vi "Note Result.vi"(8 "error in (no error)":errorcluster, 10 "Acquired Result.lvclass":refnum<class "Acquired Result.lvclass">, 11 "Measure Controller in":refnum<class "Measure Controller.lvclass">) -> (0 "error out":errorcluster, 3 "Measure Controller out":refnum<class "Measure Controller.lvclass">)   [LabVIEW 2015, in "Measure Controller.lvclass"]
uses:
  Measure Controller.lvclass
  Results/Acquired Result/Acquired Result.lvclass
  Results/Acquired Result/Acquired Result.lvclass/Acquired Result.ctl
  Measure Controller.lvclass/Measure Controller.ctl
  Results/Acquired Result/Read Sender.vi
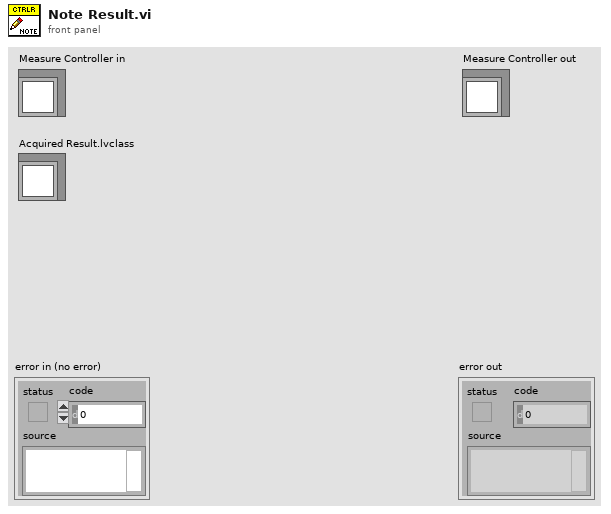
[diagram p1: front panel]
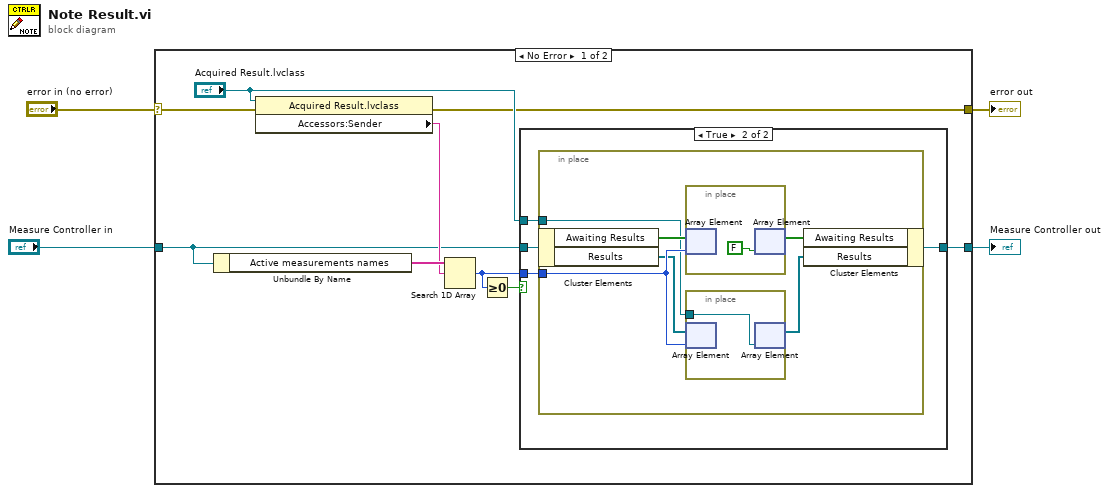
[diagram p0: block diagram]
diagram:
  n1 = case shown="No Error" "error in (no error)" {
    selector: "error in (no error)" -> [w10 w28]
    tunnel: [w9 w28] -> w3
    tunnel: [w7 w27] -> w1
    tunnel: "Measure Controller in" -> [w8 w27]
    frame No Error {
      n2 = Unbundle By Name(w8) -> ("Active measurements names"=w13:string[])
      n3 = property class="Acquired Result.lvclass"(reference="Acquired Result.lvclass", error in=w10) -> (error out=w9:errorcluster, "Accessors:Sender"=w12:string)  [unwired: 1 out]
      n4 = Search 1D Array(1D array=w13, element=w12) -> (index of element=w5:i32)  [unwired: 1 in]
      n5 = Greater Or Equal To 0?(x=w5) -> (x >= 0?=w6:bool)
      n6 = case shown="True" w6 {
        tunnel: w5 -> [_ w18]
        tunnel: "Acquired Result.lvclass" -> [_ w17]
        tunnel: w8 -> [w14 w16]
        tunnel: [w14 w15] -> w7
        frame False {
        }
        frame True {
          n7 = in-place {
            in-place-border: w18 -> [w22]
            in-place-border: w17 -> [w20]
            n8 = in-place-cluster #1(w16) -> ("Awaiting Results"=w24:bool[], "Results"=w21:refnum<class "Acquired Result.lvclass">[])
            n9 = in-place {
              n10 = in-place-array #2(w24, w22) -> ()  [unwired: 1 out]
              n11 = in-place-array #2(FALSE ("new element/subarray")) -> (w23:bool[])  [unwired: 1 out]
            }
            n12 = in-place {
              in-place-border: w20 -> [w25]
              n13 = in-place-array #3(w21, w22) -> ()  [unwired: 1 out]
              n14 = in-place-array #3(w25) -> (w19:refnum<class "Acquired Result.lvclass">[])  [unwired: 1 out]
            }
            n15 = in-place-cluster #1("Awaiting Results"=w23, "Results"=w19) -> (w15:refnum<class "Measure Controller.lvclass">)
          }
        }
      }
    }
    frame Error {
    }
  }
  "error out" <- w3
  "Measure Controller out" <- w1
